vi "VAT_valve_get_operating_mode.vi"(0 "VAT Valve COM port":refnum<visa-resource-name>, 11 "error in (no error)":errorcluster) -> (4 "VAT Valve COM port out":refnum<visa-resource-name>, 12 "Operating Mode String":string, 14 "Operating Mode":u16(ring) items=["Pressure", "Flow", "Wait"], 15 "error out":errorcluster)   [LabVIEW 2019]
uses:
  <vilib>/regexp/Match Regular Expression.xnode
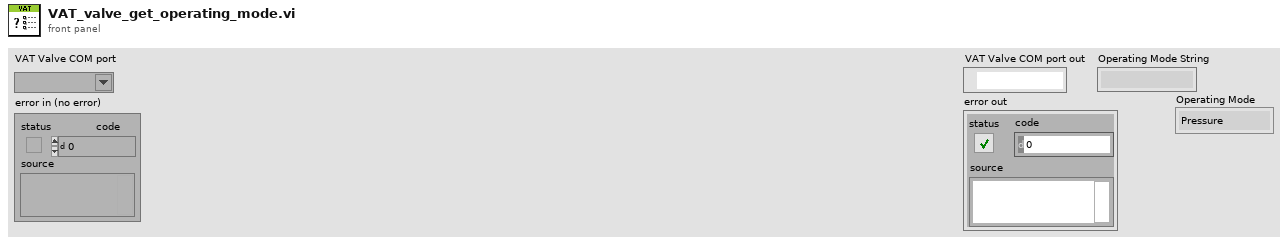
[diagram p1: front panel]
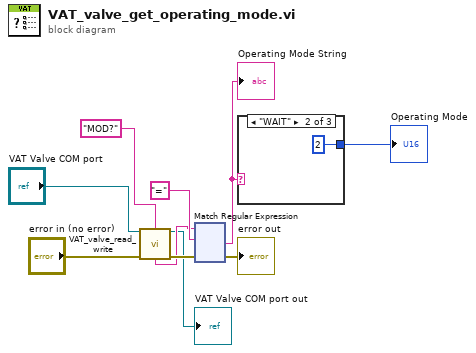
[diagram p0: block diagram]
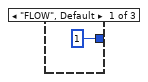
[diagram p2: hidden frame]
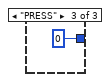
[diagram p3: hidden frame]
diagram:
  n1 = call "VAT_valve_read_write.vi"("VAT Valve COM port"="VAT Valve COM port", "Write String"="MOD?", "error in (no error)"="error in (no error)") -> ("VAT Valve COM port out"=→"VAT Valve COM port out":refnum<visa-resource-name>, "Read String"=w4:string, "error out"=w6:errorcluster)  [unwired: 10 in]
  n2 = xnode "Match Regular Expression"("input string"=w4, "regular expression"="=", "error in"=w6) -> ("after match"=w2:string, "error out"=→"error out":errorcluster)  [unwired: 3 in, 3 out]
  "Operating Mode String" <- w2
  n3 = case shown="\"WAIT\"" w2 {
    tunnel: [1 2 0] -> w1
    frame "FLOW", Default {
    }
    frame "WAIT" {
    }
    frame "PRESS" {
    }
  }
  "Operating Mode" <- w1
